vi "Read Channel with Delay.vi"(7 "milliseconds to wait":u32=1000, 8 "error in":errorcluster, 10 "Timestamp Channel":string, 11 "WorkspaceManager in":T1) -> (0 "error out":errorcluster, 1 "Delayed Value":dbl, 2 "Initial Value":dbl, 3 "WorkspaceManager out":T1)   [LabVIEW 2020, in "Loopback.lvclass"]
uses:
  Loopback.lvclass
  1d0de80c-6083-4e42-9668-24f7cee0414b.vi
  <vilib>/NI VeriStand/Execution/Workspace/NI_VS Workspace ExecutionAPI.lvlib
  <vilib>/NI VeriStand/Execution/Workspace/NI VeriStand - Get Single Channel Value.vi
  NationalInstruments.VeriStand.ClientAPI
  <vilib>/NI VeriStand/Execution/Workspace/WorkspaceAPI.ctl
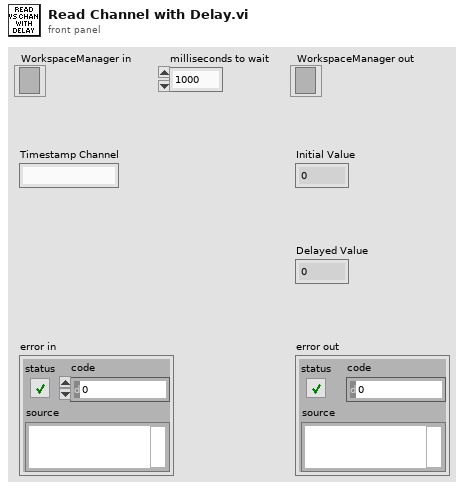
[diagram p1: front panel]
types:
  T1 = typedef "NI_VS Workspace ExecutionAPI.lvlib/WorkspaceAPI.ctl" = refnum<k24>
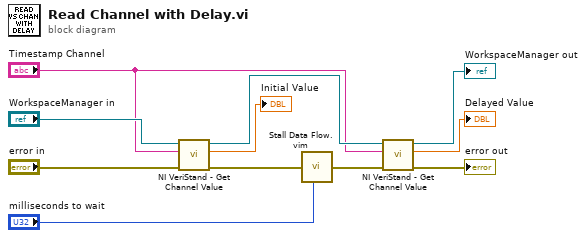
[diagram p0: block diagram]
diagram:
  n1 = call-poly <vilib>:"NI VeriStand - Get Channel Value.vi"("error in (no error)"="error in", "Channel"="Timestamp Channel", "WorkspaceManager in"="WorkspaceManager in") -> ("error out"=w7:errorcluster, "Value"=→"Initial Value":dbl, "WorkspaceManager out"=w9:T1)  [unwired: 6 in]
  n2 = call "Stall Data Flow.vim"("value in"=w7, "milliseconds to wait"="milliseconds to wait") -> ("value out"=w8:errorcluster)  [unwired: 1 out]
  n3 = call-poly <vilib>:"NI VeriStand - Get Channel Value.vi"("error in (no error)"=w8, "Channel"="Timestamp Channel", "WorkspaceManager in"=w9) -> ("error out"=→"error out":errorcluster, "Value"=→"Delayed Value":dbl, "WorkspaceManager out"=→"WorkspaceManager out":T1)  [unwired: 6 in]
